vi "Client Disconnected.vi"(8 "error in (no error)":errorcluster, 10 "GUID":string, 11 "Server Controller in":refnum<class "Server Controller.lvclass">) -> (0 "error out":errorcluster, 3 "Server Controller out":refnum<class "Server Controller.lvclass">)   [LabVIEW 2013, in "Server Controller.lvlib" / "Server Controller.lvclass"]
uses:
  Server Controller.lvclass
  Server Controller.lvclass/Server Controller.ctl
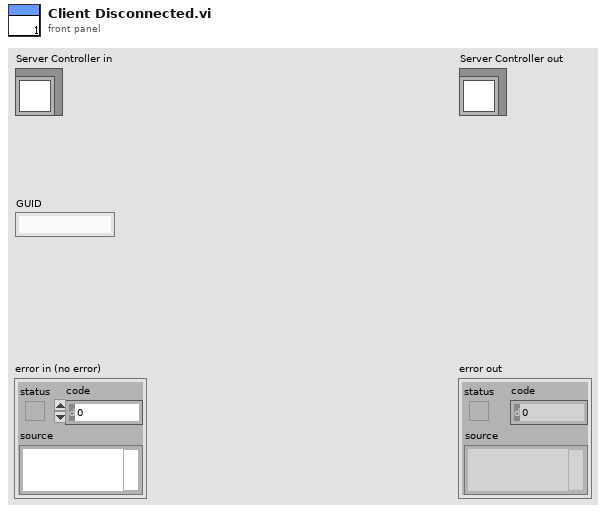
[diagram p1: front panel]
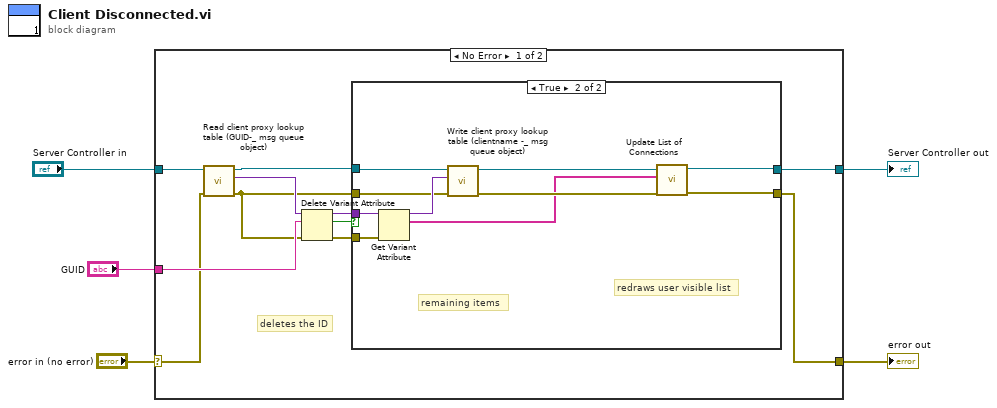
[diagram p0: block diagram]
diagram:
  n1 = case shown="No Error" "error in (no error)" {
    selector: "error in (no error)" -> [w8 w30]
    tunnel: [w6 w30] -> w4
    tunnel: [w14 w29] -> w2
    tunnel: "Server Controller in" -> [w15 w29]
    tunnel: "GUID" -> [w16 _]
    frame No Error {
      # "deletes the ID"
      n2 = call "Read client proxy lookup table (GUID-_ msg queue object).vi"("error in (no error)"=w8, "Server Controller in"=w15) -> ("error out"=w7:errorcluster, "client proxy lookup table (clientname -> msg queue object)"=w13:variant, "Server Controller out"=w12:refnum<class "Server Controller.lvclass">)  [unwired: 7 in]
      n3 = Delete Variant Attribute(4:w7, 6:w16, 7:w13) -> (0:w9:errorcluster, 2:w10:bool, 3:w11:variant)
      n4 = case shown="True" w10 {
        tunnel: w12 -> [w18 w28]
        tunnel: w11 -> [_ w27]
        tunnel: [w18 w22] -> w14
        tunnel: w9 -> [_ w25]
        tunnel: w7 -> [w17 w24]
        tunnel: [w17 w21] -> w6
        frame False {
        }
        frame True {
          # "remaining items"
          # "redraws user visible list"
          n5 = Get Variant Attribute(Variant=w27, error in=w25) -> (duplicate Variant=w26:variant, names=w19:string[])  [unwired: 2 in, 2 out]
          n6 = call "Write client proxy lookup table (clientname -_ msg queue object).vi"("error in (no error)"=w24, "client proxy lookup table (clientname -> msg queue object)"=w26, "Server Controller in"=w28) -> ("error out"=w20:errorcluster, "Server Controller out"=w23:refnum<class "Server Controller.lvclass">)  [unwired: 7 in]
          n7 = call "Update List of Connections.vi"("error in (no error)"=w20, "GUIDs"=w19, "Server Controller in"=w23) -> ("error out"=w21:errorcluster, "Server Controller out"=w22:refnum<class "Server Controller.lvclass">)  [unwired: 7 in]
        }
      }
    }
    frame Error {
    }
  }
  "error out" <- w4
  "Server Controller out" <- w2
